vi "GetAttributeViReal64_CP_Monitor_PS_Waveform.vi"(8 "error in (no error)":errorcluster {"code" format="%.0x"}, 9 "AttributeID":u32(ring)=1190234 items=["CHANNELPOWER_DISPLAY_WINDOWY_REFERENCE"=1190234, "CHANNELPOWER_DISPLAY_WINDOWY_SCALE"=1190235, "CHANNELPOWER_FILTER_ALPHA"=1190237, "CHANNELPOWER_FILTER_BANDWIDTH"=1190239, "CHANNELPOWER_FREQUENCY_SPAN"=1190240, "CHANNELPOWER_INTEGRATION_BANDWIDTH"=1150042, "CHANNELPOWER_MARKER_AMPLITUDE"=1190241, "CHANNELPOWER_MARKER_POSITION"=1190254, "CHANNELPOWER_MARKER_TRACE_POINTS_POSITION"=1190661, "CHANNELPOWER_POWER_LIMIT"=1191662, "CHANNELPOWER_PSD_LIMIT"=1191692, "CHANNELPOWER_SWEEPCOUPLING_RESOLUTION_BANDWIDTH"=1190256, "CHANNELPOWER_SWEEPCOUPLING_SWEEP_TIME"=1190259, "CHANNELPOWER_SWEEPCOUPLING_VIDEO_BANDWIDTH"=1190262, "MONITOR_DISPLAY_WINDOWY_REFERENCE"=1190352, "MONITOR_DISPLAY_WINDOWY_SCALE"=1190353, "MONITOR_FREQUENCY_SPAN_RESOLUTION_BANDWIDTH_RATIO"=1190344, "MONITOR_FREQUENCY_SPAN"=1190343, "MONITOR_MARKER_AMPLITUDE"=1190369, "MONITOR_MARKER_FUNCTION_BAND_LEFT"=1190376, "MONITOR_MARKER_FUNCTION_BAND_RIGHT"=1190377, "MONITOR_MARKER_FUNCTION_BAND_SPAN"=1190379, "MONITOR_MARKER_POSITION"=1190374, "MONITOR_MARKER_TRACE_POINTS_POSITION"=1191683, "MONITOR_SWEEPCOUPLING_RESOLUTION_BANDWIDTH"=1190360, "MONITOR_SWEEPCOUPLING_SWEEP_TIME"=1190363, "MONITOR_SWEEPCOUPLING_VIDEO_BANDWIDTH_RATIO"=1190367, "MONITOR_SWEEPCOUPLING_VIDEO_BANDWIDTH"=1190365, "POWER_STATISTICS_CHANNEL_BANDWIDTH"=1190420, "POWER_STATISTICS_DISPLAY_WINDOWX_X_SCALE"=1190434, "POWER_STATISTICS_MARKER_AMPLITUDE"=1190424, "POWER_STATISTICS_MARKER_POSITION"=1190429, "POWER_STATISTICS_MARKER_TRACE_POINTS_POSITION"=1190666, "POWER_STATISTICS_SWEEP_COUPLING_SWEEP_TIME"=1190421, "PRESELECTOR_ADJUST"=1190123, "WAVEFORM_BANDWIDTH_RESOLUTION"=1190541, "WAVEFORM_DISPLAY_IQWAVEFORM_VIEW_WINDOWX_REFERENCE"=1191575, "WAVEFORM_DISPLAY_IQWAVEFORM_VIEW_WINDOWX_SCALE"=1191576, "WAVEFORM_DISPLAY_IQWAVEFORM_VIEW_WINDOWY_REFERENCE"=1191579, "WAVEFORM_DISPLAY_IQWAVEFORM_VIEW_WINDOWY_SCALE"=1191580, "WAVEFORM_DISPLAY_WINDOWX_REFERENCE"=1190545, "WAVEFORM_DISPLAY_WINDOWX_SCALE"=1190546, "WAVEFORM_DISPLAY_WINDOWY_REFERENCE"=1190548, "WAVEFORM_DISPLAY_WINDOWY_SCALE"=1190549, "WAVEFORM_FILTER_ALPHA"=1191497, "WAVEFORM_FILTER_BANDWIDTH"=1191498, "WAVEFORM_IF_GAIN_OFFSET"=1191506, "WAVEFORM_MARKER_AMPLITUDE"=1190552, "WAVEFORM_MARKER_FUNCTION_BAND_LEFT"=1190558, "WAVEFORM_MARKER_FUNCTION_BAND_RIGHT"=1190559, "WAVEFORM_MARKER_FUNCTION_BAND_SPAN"=1190560, "WAVEFORM_MARKER_POSITION"=1190562, "WAVEFORM_MARKER_TRACE_POINTS_POSITION2"=1191573, "WAVEFORM_SAMPLE_RATE"=1191501, "WAVEFORM_SWEEP_TIME"=1190534], 10 "RepCapIdentifier":string, 11 "instrument handle":refnum<k15>) -> (0 "error out":errorcluster {"code" format="%.0x"}, 2 "AttributeValue":dbl, 3 "instrument handle out":refnum<k15>)   [LabVIEW 2021, in "Keysight XSAnVMA.lvlib"]
doc: "Gets Real64 Attribute from instrumrnt driver.\nThe following attributes are supported:\n\nCHANNELPOWER_DISPLAY_WINDOWY_REFERENCE\nCHANNELPOWER_DISPLAY_WINDOWY_SCALE\nCHANNELPOWER_FILTER_ALPHA\nCHANNELPOWER_FILTER_BANDWIDTH\nCHANNELPOWER_FREQUENCY_SPAN\nCHANNELPOWER_INTEGRATION_BANDWIDTH\nCHANNELPOWER_MARKER_AMPLITUDE\nCHANNELPOWER_MARKER_POSITION\nCHANNELPOWER_MARKER_TRACE_POINTS_POSITION\nCHANNELPOWER_POWER_LIMIT\nCHANNELPOWER_PSD_LIMIT\nCHANNELPOWER_SWEEPCOUPLING_RESOLUTION_BANDWIDTH\nCHANNELPOWER_SWEEPCOUPLING_SWEEP_TIME\nCHANNELPOWER_SWEEPCOUPLING_VIDEO_BANDWIDTH\nMONITOR_DISPLAY_WINDOWY_REFERENCE\nMONITOR_DISPLAY_WINDOWY_SCALE\nMONITOR_FREQUENCY_SPAN_RESOLUTION_BANDWIDTH_RATIO\nMONITOR_FREQUENCY_SPAN\nMONITOR_MARKER_AMPLITUDE\nMONITOR_MARKER_FUNCTION_BAND_LEFT\nMONITOR_MARKER_FUNCTION_BAND_RIGHT\nMONITOR_MARKER_FUNCTION_BAND_SPAN\nMONITOR_MARKER_POSITION\nMONITOR_MARKER_TRACE_POINTS_POSITION\nMONITOR_SWEEPCOUPLING_RESOLUTION_BANDWIDTH\nMONITOR_SWEEPCOUPLING_SWEEP_TIME\nMONITOR_SWEEPCOUPLING_VIDEO_BANDWIDTH_RATIO\nMONITOR_SWEEPCOUPLING_VIDEO_BANDWIDTH\nPOWER_STATISTICS_CHANNEL_BANDWIDTH\nPOWER_STATISTICS_DISPLAY_WINDOWX_X_SCALE\nPOWER_STATISTICS_MARKER_AMPLITUDE\nPOWER_STATISTICS_MARKER_POSITION\nPOWER_STATISTICS_MARKER_TRACE_POINTS_POSITION\nPOWER_STATISTICS_SWEEP_COUPLING_SWEEP_TIME\nPRESELECTOR_ADJUST\nWAVEFORM_BANDWIDTH_RESOLUTION\nWAVEFORM_DISPLAY_IQWAVEFORM_VIEW_WINDOWX_REFERENCE\nWAVEFORM_DISPLAY_IQWAVEFORM_VIEW_WINDOWX_SCALE\nWAVEFORM_DISPLAY_IQWAVEFORM_VIEW_WINDOWY_REFERENCE\nWAVEFORM_DISPLAY_IQWAVEFORM_VIEW_WINDOWY_SCALE\nWAVEFORM_DISPLAY_WINDOWX_REFERENCE\nWAVEFORM_DISPLAY_WINDOWX_SCALE\nWAVEFORM_DISPLAY_WINDOWY_REFERENCE\nWAVEFORM_DISPLAY_WINDOWY_SCALE\nWAVEFORM_FILTER_ALPHA\nWAVEFORM_FILTER_BANDWIDTH\nWAVEFORM_IF_GAIN_OFFSET\nWAVEFORM_MARKER_AMPLITUDE\nWAVEFORM_MARKER_FUNCTION_BAND_LEFT\nWAVEFORM_MARKER_FUNCTION_BAND_RIGHT\nWAVEFORM_MARKER_FUNCTION_BAND_SPAN\nWAVEFORM_MARKER_POSITION\nWAVEFORM_MARKER_TRACE_POINTS_POSITION2\nWAVEFORM_SAMPLE_RATE\nWAVEFORM_SWEEP_TIME"
uses:
  <instrlib>/Keysight XSAnVMA/Keysight XSAnVMA.lvlib
  KtXSAnVMA_64.dll
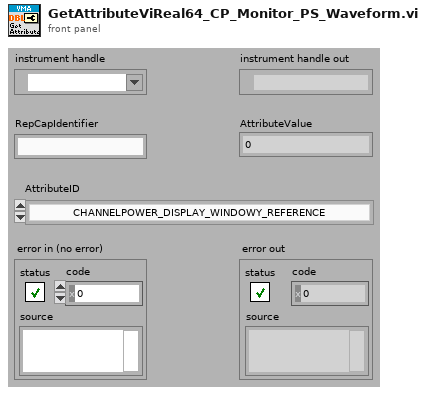
[diagram p1: front panel]
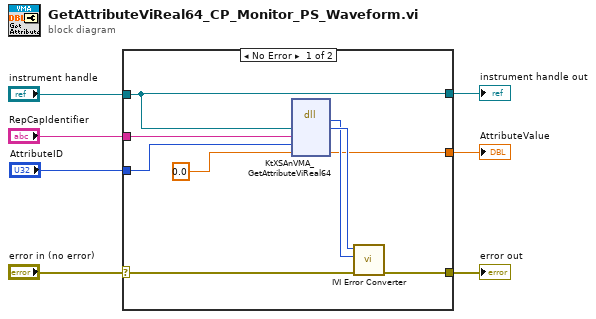
[diagram p0: block diagram]
diagram:
  n1 = case shown="No Error" "error in (no error)" {
    selector: "error in (no error)" -> [w14 w18]
    tunnel: [w13 w18] -> w7
    tunnel: "instrument handle" -> [w8 w17]
    tunnel: "RepCapIdentifier" -> [w12 _]
    tunnel: "AttributeID" -> [w11 _]
    tunnel: [w9 _] -> w3
    tunnel: [w8 w17] -> w2
    frame No Error {
      n2 = dll-call lib="KtXSAnVMA**.dll" fn="KtXSAnVMA_GetAttributeViReal64"("Vi"=w8, "RepCapIdentifier"=w12, "AttributeID"=w11, "AttributeValue"=0.0) -> ("return type"=w15:i32, "Vi"=w16:u32, "AttributeValue"=w9:dbl)  [unwired: 5 in, 2 out]
      n3 = call <instrlib>:"IVI Error Converter.vi"("error in (no error)"=w14, "IVI error code (0)"=w15, "instrument handle"=w16) -> ("error out"=w13:errorcluster)  [unwired: 7 in, 1 out]
    }
    frame Error {
    }
  }
  "error out" <- w7
  "instrument handle out" <- w2
  "AttributeValue" <- w3
